vi "Update_UI.vi"(8 "error in (no error)":errorcluster, 10 "srcsettings":T1, 11 "IB_Settings_Item in":refnum<class "IB_Settings_Item.lvclass">) -> (0 "error out":errorcluster, 2 "validate permisions?":bool, 3 "IB_Settings_Item out":refnum<class "IB_Settings_Item.lvclass">)   [LabVIEW 2020, in "IB_Settings_Item.lvclass"]
uses:
  <vilib>/AppBuilder/IB_Classes/Settings_Item/IB_Settings_Item.lvclass
  <vilib>/AppBuilder/IB_Classes/Settings_Item/IB_Settings_Item.lvclass/IB_Settings_Item.ctl
  <resource>/Framework/Providers/Builds/Installer/CDK_sTypeDef_FILEATTRIBUTES.ctl
  <resource>/Framework/Providers/Builds/Installer/Pages/controls/IB_UI_Page_SrcSettings_References.ctl
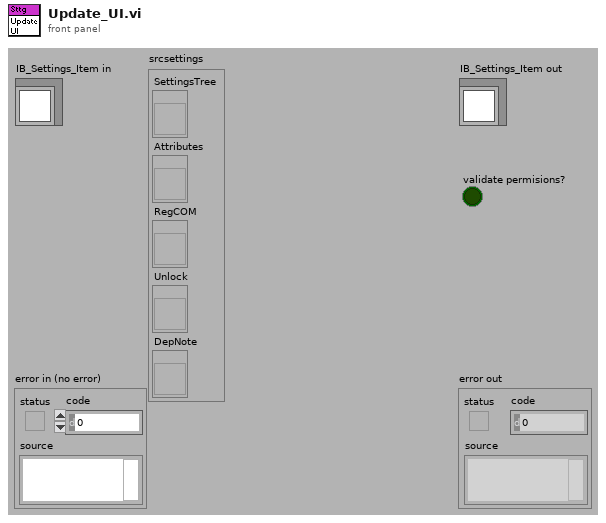
[diagram p1: front panel]
types:
  T1 = typedef "IB_UI_Page_SrcSettings_References.ctl" = cluster{"SettingsTree":refnum<vi>, "Attributes":refnum<vi>, "RegCOM":refnum<vi>, "Unlock":refnum<vi>, "DepNote":refnum<vi>}
  T2 = typedef "CDK_sTypeDef_FILEATTRIBUTES.ctl" = cluster{"fAttribute":bool, "fAttribute 2":bool, "fAttribute 3":bool, "fAttribute 4":bool}
  T3 = enum8{"Enabled", "Disabled", "Disabled and Grayed Out"}
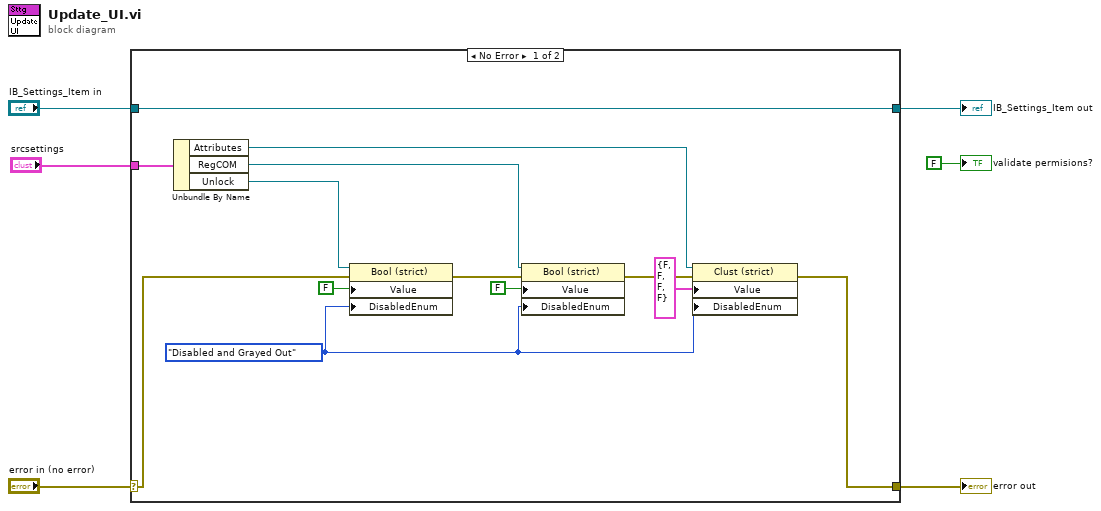
[diagram p0: block diagram]
diagram:
  n1 = case shown="No Error" "error in (no error)" {
    selector: "error in (no error)" -> [w7 w21]
    tunnel: [w8 w21] -> w5
    tunnel: [w19 w20] -> w3
    tunnel: "IB_Settings_Item in" -> [w19 w20]
    tunnel: "srcsettings" -> [w18 _]
    frame No Error {
      w13 = T3."Disabled and Grayed Out" ("Disabled")
      n2 = Unbundle By Name(w18) -> ("Attributes"=w15:refnum<vi>, "RegCOM"=w16:refnum<vi>, "Unlock"=w17:refnum<vi>)
      n3 = property class="Bool (strict)"(reference=w17, error in=w7, "Value"=FALSE, "DisabledEnum"=w13) -> (error out=w10:errorcluster)  [unwired: 1 out]
      n4 = property class="Bool (strict)"(reference=w16, error in=w10, "Value"=FALSE, "DisabledEnum"=w13) -> (error out=w9:errorcluster)  [unwired: 1 out]
      n5 = property class="Clust (strict)"(reference=w15, error in=w9, "Value"=T2 {"fAttribute"=FALSE, "fAttribute 2"=FALSE, "fAttribute 3"=FALSE, "fAttribute 4"=FALSE}, "DisabledEnum"=w13) -> (error out=w8:errorcluster)  [unwired: 1 out]
    }
    frame Error {
    }
  }
  "error out" <- w5
  "IB_Settings_Item out" <- w3
  "validate permisions?" <- FALSE ("validate permisions?")
